vi "Stop Core.vi"(10 "final error code":i32, 11 "Mag Lab Measure Controller in":refnum<class "Mag Lab Measure Controller.lvclass">) -> (3 "Mag Lab Measure Controller out":refnum<class "Mag Lab Measure Controller.lvclass">)   [LabVIEW 2015, in "Mag Lab Measure Controller.lvclass"]
uses:
  Mag Lab Measure Controller.lvclass
  Mag Lab Measure Controller.lvclass/Mag Lab Measure Controller.ctl
  <vilib>/ActorFramework/Message Enqueuer/Message Enqueuer.lvclass/Message Enqueuer.ctl
  <vilib>/ActorFramework/Message Enqueuer/Enqueue.vi
  <vilib>/ActorFramework/Message Priority Queue/Priority Enqueue.vi
  <vilib>/ActorFramework/Stop Msg/Stop Msg.lvclass
  Compound Measurement/Compound Measurement.lvclass
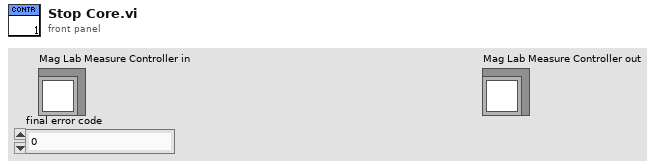
[diagram p1: front panel]
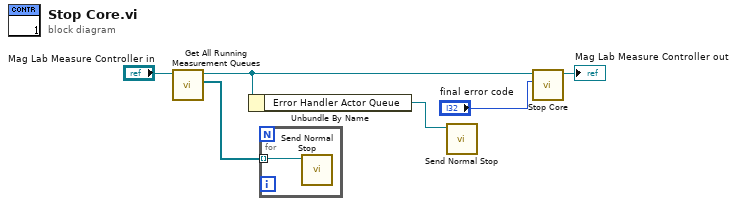
[diagram p0: block diagram]
diagram:
  n1 = call "Get All Running Measurement Queues.vi"("Mag Lab Measure Controller in"="Mag Lab Measure Controller in") -> ("Array of Measurement Queues"=w3:refnum<class "Message Enqueuer.lvclass">[], "Mag Lab Measure Controller out"=w2:refnum<class "Mag Lab Measure Controller.lvclass">)  [unwired: 8 in, 1 out]
  n2 = Unbundle By Name(w2) -> ("Error Handler Actor Queue"=w1:refnum<class "Message Enqueuer.lvclass">)
  n3 = for {
    tunnel: w3 -> [w7] mode=indexing
    n4 = call <vilib>:"Send Normal Stop.vi"("Message Enqueuer"=w7) -> ()  [unwired: 10 in, 1 out]
  }
  n5 = call <vilib>:"Send Normal Stop.vi"("Message Enqueuer"=w1) -> ()  [unwired: 10 in, 1 out]
  n6 = call-parent "Stop Core.vi"("final error code"="final error code", "Mag Lab Measure Base in"=w2) -> ("Mag Lab Measure Base out"=→"Mag Lab Measure Controller out":refnum<class "Mag Lab Measure Controller.lvclass">)  [unwired: 9 in]
